vi "Subscriber.vi"(9 "OpenWindow":bool, 10 "endpoint":string="tcp://192.168.3.98:55555", 11 "stop 2":bool) -> ()   [LabVIEW 2014]
uses:
  lvnanomsg/nanomsg_context.lvclass
  lvnanomsg/nanomsg_socket.lvclass
panel:
  out "Numeric":u64
  out "dT":u32
  out "Waveform Chart":dbl(graph)
  out "error IO":errorcluster
  in  "stop":bool
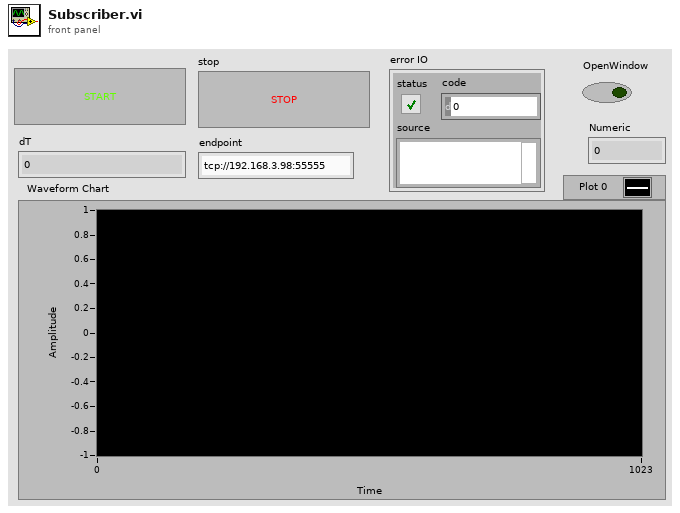
[diagram p1: front panel]
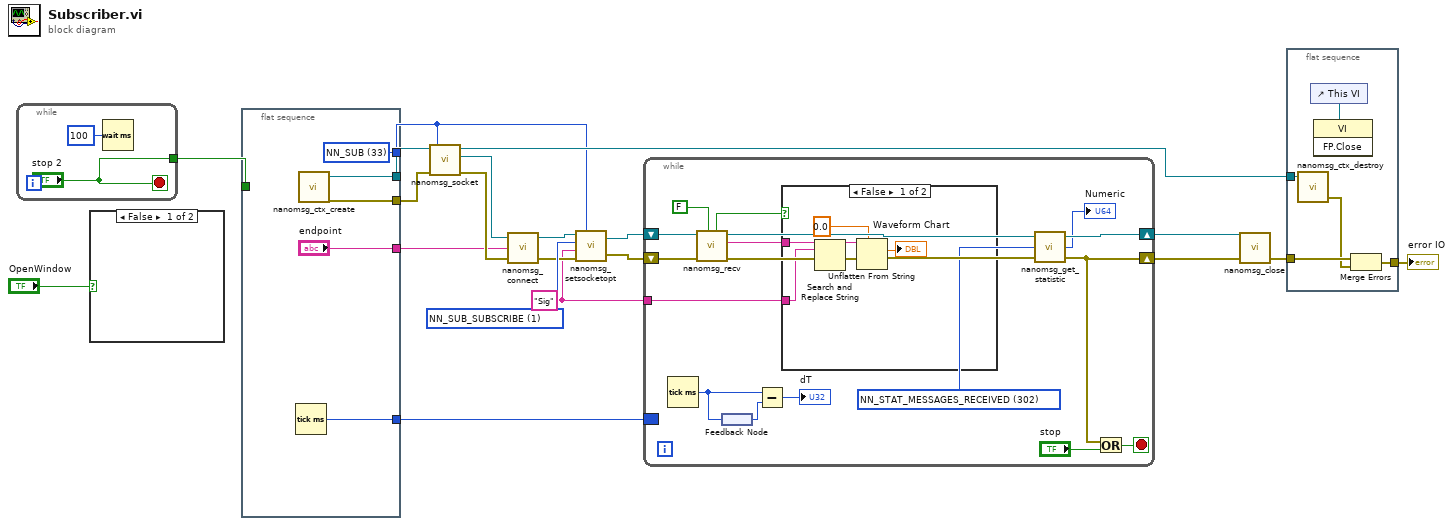
[diagram p0: block diagram]
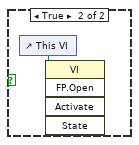
[diagram p2: hidden frame]
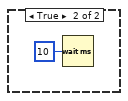
[diagram p3: hidden frame]
diagram:
  w5 = "Sig" ("data 2")
  w13 = 1 items=["NN_SUB_SUBSCRIBE"=1, "NN_SUB_UNSUBSCRIBE"=2] ("option")
  n1 = while {
    tunnel: ["stop 2"] -> w14
    stop <- "stop 2" stop-if-true
    n2 = Wait (ms)(milliseconds to wait=u32 100) -> ()  [unwired: 1 out]
  }
  n3 = case shown="False" "OpenWindow" {
    frame False {
    }
    frame True {
      n4 = control-ref of="This VI"() -> (w23:refnum<vi>)
      n5 = invoke class="VI" method="FP.Open"(reference=w23) -> ()  [unwired: 4 in, 5 out]
    }
  }
  n6 = flat-sequence {
    tunnel: [w28] -> w20
    tunnel: [w27] -> w19
    tunnel: [w26] -> w1
    tunnel: ["endpoint"] -> w8
    tunnel: w14 -> [_]
    tunnel: [w24] -> w4
    frame #0 {
      w26 = 33 items=["NN_WS"=-4, "NN_TCP"=-3, "NN_IPC"=-2, "NN_INPROC"=-1, "NN_SOL_SOCKET"=0, "NN_PAIR"=16, "NN_PUB"=32, "NN_SUB"=33, "NN_REQ"=48, "NN_REP"=49, "NN_PUSH"=80, "NN_PULL"=81, "NN_SURVEYOR"=98, "NN_RESPONDENT"=99, "NN_BUS"=112] ("socket type")
      n7 = Tick Count (ms)() -> (millisecond timer value=w24:u32)
      n8 = call "nanomsg_ctx_create.vi"() -> ("error out"=w27:errorcluster, "context out"=w28:refnum<class "nanomsg_context.lvclass">)  [unwired: 4 in]
    }
  }
  n9 = call "nanomsg_socket.vi"("error in"=w19, "socket type"=w1, "context in"=w20) -> ("error out"=w15:errorcluster, "socket out"=w16:refnum<class "nanomsg_socket.lvclass">, "context out"=w2:refnum<class "nanomsg_context.lvclass">)  [unwired: 2 in]
  n10 = call "nanomsg_connect.vi"("error in"=w15, "endpoint"=w8, "socket in"=w16) -> ("error out"=w10:errorcluster, "socket out"=w12:refnum<class "nanomsg_socket.lvclass">)  [unwired: 1 in]
  n11 = call "nanomsg_setsocketopt.vi"("socket in"=w12, "option"=w13, "value"=w5, "error in"=w10, "level"=w1) -> ("socket out"=w11:refnum<class "nanomsg_socket.lvclass">, "error out"=w9:errorcluster)
  n12 = while {
    shift-right: [w33] -> w7
    shift-left: w11 -> [w43]
    shift-right: [w31] -> w6
    shift-left: w9 -> [w42]
    tunnel: w5 -> [w39]
    border: w4 -> [_]
    stop <- w44 stop-if-true
    w30 = 302 items=["NN_STAT_ESTABLISHED_CONNECTIONS"=101, "NN_STAT_ACCEPTED_CONNECTIONS"=102, "NN_STAT_DROPPED_CONNECTIONS"=103, "NN_STAT_BROKEN_CONNECTIONS"=104, "NN_STAT_CONNECT_ERRORS"=105, "NN_STAT_BIND_ERRORS"=106, "NN_STAT_ACCEPT_ERRORS"=107, "NN_STAT_CURRENT_CONNECTIONS"=201, "NN_STAT_INPROGRESS_CONNECTIONS"=202, "NN_STAT_CURRENT_EP_ERRORS"=203, "NN_STAT_MESSAGES_SENT"=301, "NN_STAT_MESSAGES_RECEIVED"=302, "NN_STAT_BYTES_SENT"=303, "NN_STAT_BYTES_RECEIVED"=304, "NN_STAT_CURRENT_SND_PRIORITY"=401] ("statistics type")
    n13 = Tick Count (ms)() -> (millisecond timer value=w36:u32)
    n14 = call "nanomsg_recv.vi"("no block? (F)"=FALSE, "error in"=w42, "socket in"=w43) -> ("error out"=w32:errorcluster, "data"=w40:string, "socket out"=w41:refnum<class "nanomsg_socket.lvclass">, "timeout?"=w37:bool)  [unwired: 2 in, 1 out]
    n15 = feedback-in #1(w36) -> ()
    n16 = feedback #1() -> (w35:u32)
    n17 = Subtract(x=w36, y=w35) -> (x-y=→"dT":u32)
    n18 = case shown="False" w37 {
      tunnel: w40 -> [w50 _]
      tunnel: w39 -> [w49 _]
      frame False {
        n19 = Search and Replace String(input string=w50, search string=w49) -> (result string=w48:string)  [unwired: 6 in, 3 out]
        n20 = Unflatten From String(type=0.0, binary string=w48) -> (value=→"Waveform Chart":dbl)  [unwired: 3 in, 2 out]
      }
      frame True {
        n21 = Wait (ms)(milliseconds to wait=u32 10) -> ()  [unwired: 1 out]
      }
    }
    n22 = call "nanomsg_get_statistic.vi"("error in"=w32, "statistic"=w30, "socket in"=w41) -> ("error out"=w31:errorcluster, "result"=→"Numeric":u64, "socket out"=w33:refnum<class "nanomsg_socket.lvclass">)
    n23 = Or(x=w31, y="stop") -> (x .or. y?=w44:bool)
  }
  n24 = call "nanomsg_close.vi"("error in"=w6, "socket"=w7) -> ("error out"=w18:errorcluster)  [unwired: 3 in]
  n25 = flat-sequence {
    tunnel: w2 -> [w56]
    tunnel: w18 -> [w55]
    tunnel: [w53] -> w17
    frame #0 {
      n26 = call "nanomsg_ctx_destroy.vi"("context in"=w56) -> ("error out"=w54:errorcluster)  [unwired: 4 in]
      n27 = control-ref of="This VI"() -> (w52:refnum<vi>)
      n28 = invoke class="VI" method="FP.Close"(reference=w52) -> ()  [unwired: 2 in, 3 out]
      n29 = Merge Errors(w55, w54) -> (w53:errorcluster)
    }
  }
  "error IO" <- w17
